vi "register_instance.vi"(8 "error in (no error)":errorcluster, 9 "Object Instance":refnum<data-value>, 10 "Base Class (LabVIEW Object)":refnum<class>, 11 "Default Lookup in":refnum<class "Default Lookup.lvclass">) -> (0 "error out":errorcluster, 3 "Default Lookup out":refnum<class "Default Lookup.lvclass">)   [LabVIEW 2014, in "LVCOOOP.lvlib" / "Lookup API.lvlib" / "Default Lookup.lvclass"]
doc: "Associate an object instance with the specified base class."
uses:
  Default Lookup.lvclass
  Default Lookup.lvclass/Default Lookup.ctl
  types/lookup_data.ctl
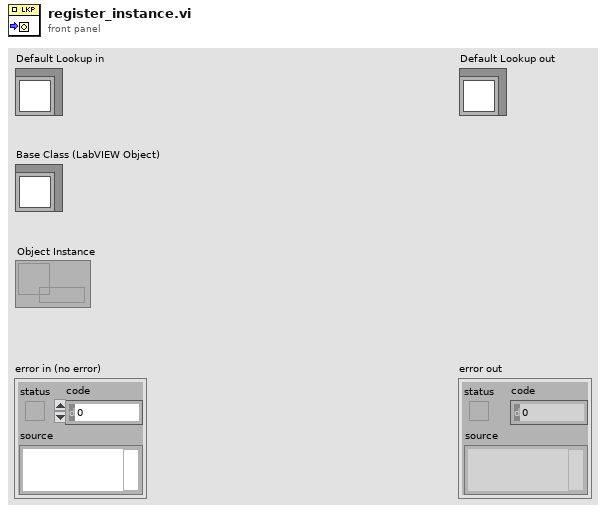
[diagram p1: front panel]
types:
  T1 = typedef "LVCOOOP.lvlib/Lookup API.lvlib/Default Lookup.lvclass/lookup_data.ctl" = cluster{"instances":refnum<data-value>[], "listeners":refnum<user-event>[]}
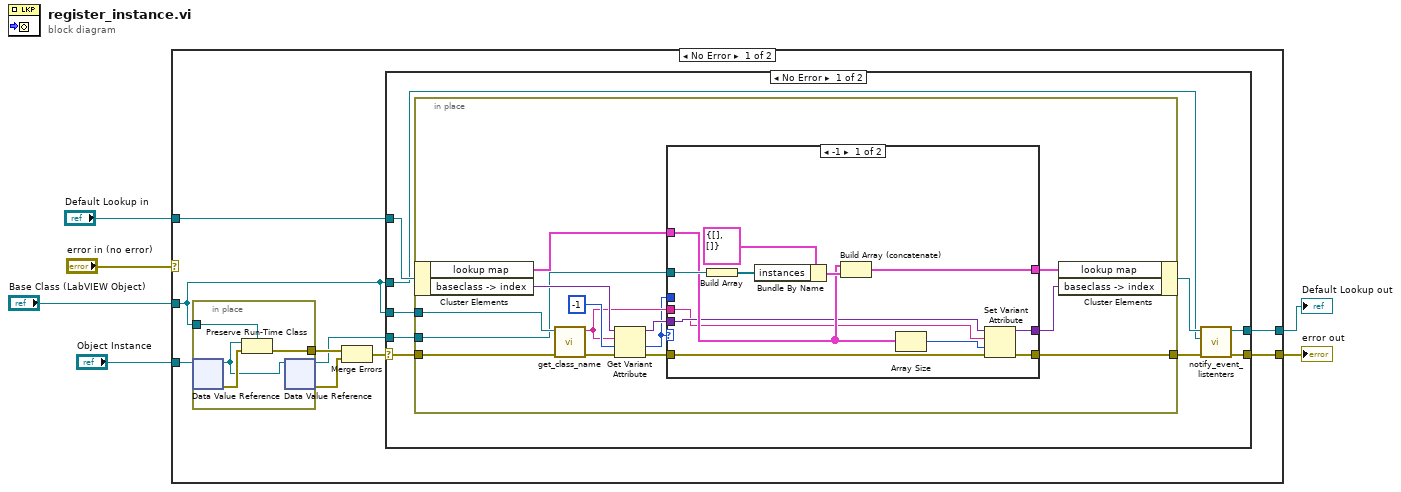
[diagram p0: block diagram]
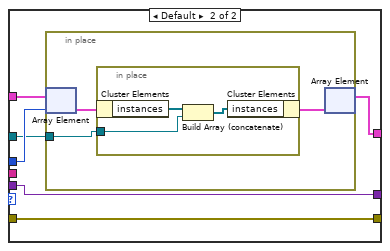
[diagram p2: hidden frame]
diagram:
  n1 = case shown="No Error" "error in (no error)" {
    selector: "error in (no error)" -> [_ w70]
    tunnel: [w8 w70] -> w5
    tunnel: "Object Instance" -> [w15 _]
    tunnel: "Base Class (LabVIEW Object)" -> [w7 _]
    tunnel: "Default Lookup in" -> [w11 w69]
    tunnel: [w9 w69] -> w1
    frame No Error {
      n2 = in-place {
        in-place-border: w7 -> [w68]
        in-place-border: [w66] -> w14
        n3 = in-place-dvr #1(w15) -> (w65:refnum<class>, w67:errorcluster)
        n4 = Preserve Run-Time Class(object in=w65, error in=w67, 2:w68) -> (error out=w66:errorcluster)  [unwired: 1 out]
        n5 = in-place-dvr #1(w65) -> (w10:refnum<data-value>, w13:errorcluster)
      }
      n6 = Merge Errors(w14, w13) -> (w12:errorcluster)
      n7 = case shown="No Error" w12 {
        selector: w12 -> [w22 w63]
        tunnel: w11 -> [w24 w64]
        tunnel: w7 -> [w23 _]
        tunnel: w10 -> [w21 _]
        tunnel: [w17 w64] -> w9
        tunnel: [w18 w63] -> w8
        tunnel: w7 -> [w16 _]
        frame No Error {
          n8 = in-place {
            in-place-border: w23 -> [w37]
            in-place-border: w22 -> [w36]
            in-place-border: w21 -> [w32]
            in-place-border: [w25] -> w19
            n9 = in-place-cluster #2(w24) -> ("lookup map"=w33:T1[], "baseclass -> index"=w38:variant)
            n10 = call "get_class_name.vi"("error in (no error)"=w36, "LabVIEW Object in"=w37) -> ("error out"=w35:errorcluster, "class name"=w29:string)  [unwired: 8 in]
            n11 = Get Variant Attribute(Variant=w38, name=w29, default value (empty Variant)=-1, error in=w35) -> (duplicate Variant=w30:variant, value=w26:i32, error out=w28:errorcluster)  [unwired: 1 out]
            n12 = case shown="-1" w26 {
              tunnel: w33 -> [w45 w56]
              tunnel: w32 -> [w49 w53]
              tunnel: [w46 w55] -> w31
              tunnel: w30 -> [w44 w52]
              tunnel: w29 -> [w43 _]
              tunnel: w28 -> [w41 w51]
              tunnel: [w40 w52] -> w27
              tunnel: w26 -> [_ w54]
              tunnel: [w39 w51] -> w25
              frame -1 {
                n13 = Build Array(w49) -> (w48:refnum<data-value>[])
                n14 = Bundle By Name(cluster=T1 {"instances"=[], "listeners"=[]} ("lookup data"), "instances"=w48) -> (w47:T1)
                n15 = Build Array (concatenate)(w45, w47) -> (w46:T1[])
                n16 = Array Size(array=w45) -> (size(s)=w42:i32)
                n17 = Set Variant Attribute(Variant=w44, name=w43, value=w42, error in=w41) -> (Variant out=w40:variant, error out=w39:errorcluster)  [unwired: 1 out]
              }
              frame Default {
                n18 = in-place {
                  in-place-border: w53 -> [w57]
                  n19 = in-place-array #3(w56, w54) -> (w59:T1)
                  n20 = in-place {
                    in-place-border: w57 -> [w60]
                    n21 = in-place-cluster #4(w59) -> ("instances"=w62:refnum<data-value>[])
                    n22 = Build Array (concatenate)(w62, w60) -> (w61:refnum<data-value>[])
                    n23 = in-place-cluster #4("instances"=w61) -> (w58:T1)
                  }
                  n24 = in-place-array #3(w58) -> (w55:T1[])  [unwired: 1 out]
                }
              }
            }
            n25 = in-place-cluster #2("lookup map"=w31, "baseclass -> index"=w27) -> (w20:refnum<class "Default Lookup.lvclass">)
          }
          n26 = call-dynamic "notify_event_listenters.vi"("error in (no error)"=w19, "Base Class (LabVIEW Object)"=w16, "Default Lookup in"=w20) -> ("error out"=w18:errorcluster, "Default Lookup out"=w17:refnum<class "Default Lookup.lvclass">)  [unwired: 7 in]
        }
        frame Error {
        }
      }
    }
    frame Error {
    }
  }
  "error out" <- w5
  "Default Lookup out" <- w1
